vi "5feladat.vi"() -> ()   [LabVIEW 2016]
panel:
  out "Boolean":bool
  out "Numeric 2":dbl
  in  "OK Button":bool
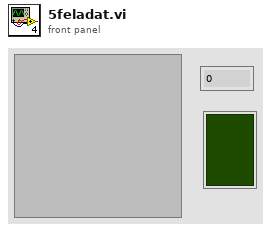
[diagram p1: front panel]
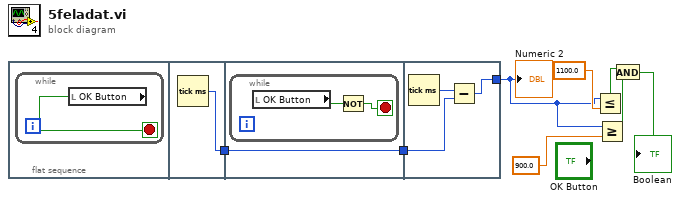
[diagram p0: block diagram]
diagram:
  n1 = flat-sequence {
    tunnel: [w10] -> w6
    tunnel: w6 -> [w11]
    tunnel: [w11] -> w5
    tunnel: w5 -> [w15]
    tunnel: [w14] -> w1
    frame #0 {
      n2 = while {
        stop <- w9 stop-if-true
        n3 = local read "OK Button"() -> (w9:bool)
      }
    }
    frame #1 {
      n4 = Tick Count (ms)() -> (millisecond timer value=w10:u32)
    }
    frame #2 {
      n5 = while {
        stop <- w12 stop-if-true
        n6 = local read "OK Button"() -> (w13:bool)
        n7 = Not(x=w13) -> (.not. x?=w12:bool)
      }
    }
    frame #3 {
      n8 = Tick Count (ms)() -> (millisecond timer value=w16:u32)
      n9 = Subtract(x=w16, y=w15) -> (x-y=w14:u32)
    }
  }
  n10 = Less Or Equal?(x=w1, y=1100.0) -> (x <= y?=w8:bool)
  n11 = Greater Or Equal?(x=w1, y=900.0) -> (x >= y?=w7:bool)
  n12 = And(x=w8, y=w7) -> (x .and. y?=→"Boolean":bool)
  "Numeric 2" <- w1
